vi "get unique channel name.vi"(8 "error in":errorcluster, 9 "prefix":string, 10 "scale name":string, 11 "channels":refnum<class "TBM channel.lvclass">[](array[class])) -> (0 "error out":errorcluster, 3 "name":string)   [LabVIEW 2013, in "Scaling configuration.lvclass"]
uses:
  Scaling configuration.lvclass
  <vilib>/NI/Tag Bus Module Framework/channel/TBM channel.lvclass
  <vilib>/NI/Tag Bus/tag/tag descriptor.lvclass/tag descriptor.ctl
  <vilib>/NI/Tag Bus/tag/tag descriptor.lvclass
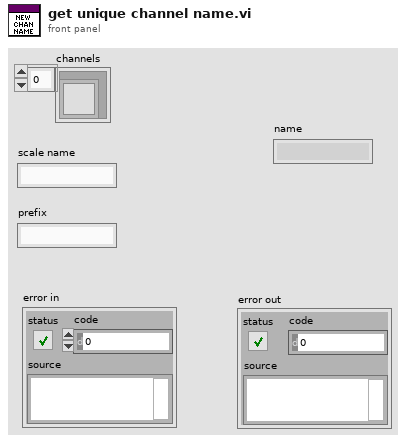
[diagram p1: front panel]
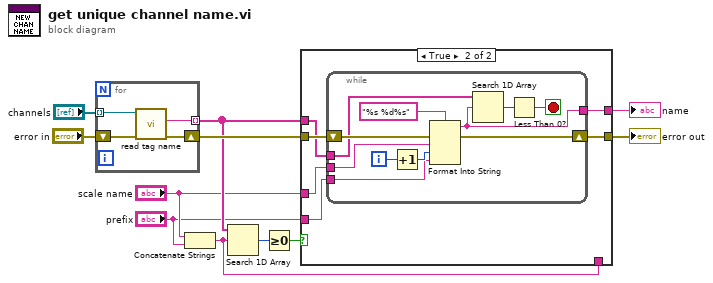
[diagram p0: block diagram]
diagram:
  n1 = for {
    tunnel: "channels" -> [w15] mode=indexing
    tunnel: [w14] -> w6 mode=indexing
    shift-right: [w13] -> w9
    shift-left: "error in" -> [w12]
    n2 = call <vilib>:"read tag name.vi"("error in"=w12, "system tag in"=w15) -> ("error out"=w13:errorcluster, "name"=w14:string)  [unwired: 7 in, 1 out]
  }
  n3 = Concatenate Strings("scale name", "prefix") -> (w1:string)
  n4 = Search 1D Array(1D array=w6, element=w1) -> (index of element=w5:i32)  [unwired: 1 in]
  n5 = Greater Or Equal To 0?(x=w5) -> (x >= 0?=w4:bool)
  n6 = case shown="True" w4 {
    tunnel: "scale name" -> [_ w19]
    tunnel: [w16 w23] -> w10
    tunnel: w6 -> [_ w20]
    tunnel: w9 -> [w17 w22]
    tunnel: [w17 w21] -> w8
    tunnel: "prefix" -> [_ w18]
    tunnel: w1 -> [w16 _]
    frame False {
    }
    frame True {
      n7 = while {
        tunnel: [w29] -> w23
        shift-right: [w27] -> w21
        shift-left: w22 -> [w28]
        tunnel: w20 -> [w26]
        tunnel: w19 -> [w25]
        tunnel: w18 -> [w24]
        i -> [w33]
        stop <- w30 stop-if-true
        n8 = Increment(x=w33) -> (x+1=w32:i32)
        n9 = Format Into String(format string="%s %d%s", error in=w28, w25, w32, w24) -> (resulting string=w29:string, error out=w27:errorcluster)  [unwired: 1 in]
        n10 = Search 1D Array(1D array=w26, element=w29) -> (index of element=w31:i32)  [unwired: 1 in]
        n11 = Less Than 0?(x=w31) -> (x < 0?=w30:bool)
      }
    }
  }
  "name" <- w10
  "error out" <- w8
